vi "welcomewindow.vi"() -> ()   [LabVIEW 2013]
panel:
  in  "stop":bool
  out "String":string
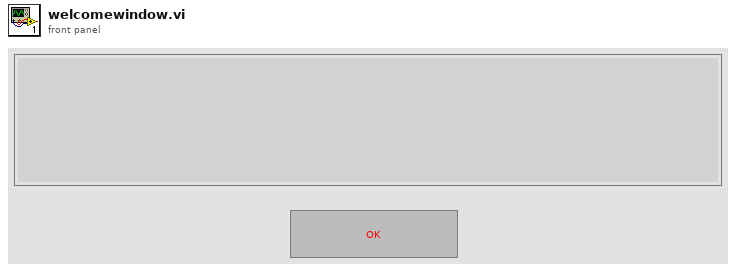
[diagram p1: front panel]
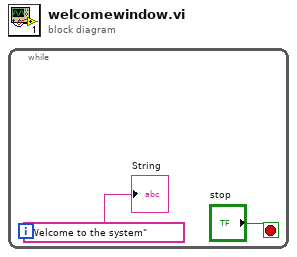
[diagram p0: block diagram]
diagram:
  n1 = while {
    stop <- "stop" stop-if-true
    "String" <- "Welcome to the system" ("String")
  }
